vi "Obtain Tree Manager.vi"(8 "Error In":errorcluster) -> (0 "Error Out":errorcluster, 3 "Tree":refnum<data-value>)   [LabVIEW 2017, in "Tree API.lvlib" / "Tree.lvclass"]
doc: "Obtain a reference to the Tree Manager. If this is the first reference initialize the Manager."
uses:
  Tree.lvclass
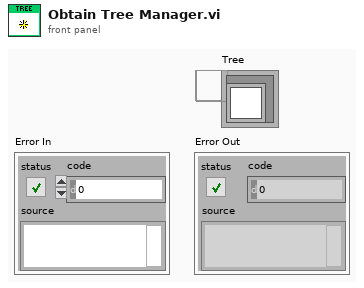
[diagram p1: front panel]
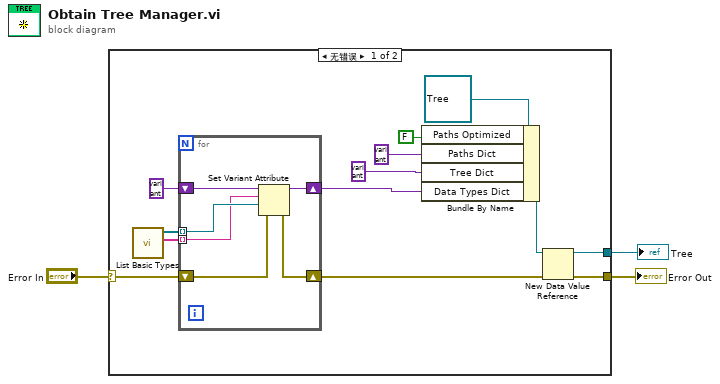
[diagram p0: block diagram]
diagram:
  n1 = case shown="无错误" "Error In" {
    selector: "Error In" -> [w11 w23]
    tunnel: [w7 w23] -> w2
    tunnel: [w8 _] -> w3
    frame No Error {
      n2 = call "List Basic Types.vi"() -> ("Long Class Names"=w4:string[], "Basic Types"=w12:refnum<class "Tree Data.lvclass">[])  [unwired: 9 in, 1 out]
      n3 = for {
        shift-right: [w21] -> w14
        shift-left: variant ("Tree Dictionary") -> [w22]
        tunnel: w12 -> [w20] mode=indexing
        shift-right: [w19] -> w10
        shift-left: w11 -> [w18]
        tunnel: w4 -> [w17] mode=indexing
        n4 = Set Variant Attribute(Variant=w22, name=w17, value=w20, error in=w18) -> (Variant out=w21:variant, error out=w19:errorcluster)  [unwired: 1 out]
      }
      n5 = Bundle By Name(cluster=refnum<class "Tree.lvclass"> refnum, "Paths Optimized"=FALSE, "Paths Dict"=variant ("Names Dict"), "Tree Dict"=variant ("Tree Dictionary"), "Data Types Dict"=w14) -> (w9:refnum<class "Tree.lvclass">)
      n6 = New Data Value Reference(data value=w9, error in=w10) -> (data value reference=w8:refnum<data-value>, error out=w7:errorcluster)
    }
    frame Error {
    }
  }
  "Tree" <- w3
  "Error Out" <- w2
